vi "Init.vi"(8 "error in (no error)":errorcluster, 9 "Value":string, 10 "Data [value]":T1=enum."value") -> (0 "error out":errorcluster, 3 "Set Query out":refnum<class "Set Query.lvclass">)   [LabVIEW 2013, in "Set Query.lvclass"]
doc: "Copyright 2018, Carya Automatisering, Wiebe Walstra."
uses:
  Set Query.lvclass
  Data.ctl
  Set Query.lvclass/Set Query.ctl
  CConfig Object.lvclass
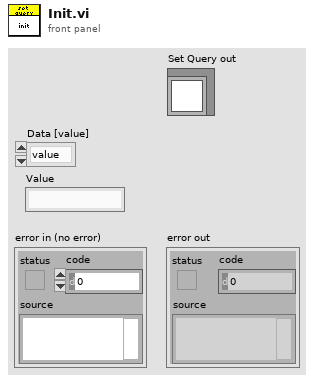
[diagram p1: front panel]
types:
  T1 = typedef "CConfig Object.lvclass/Data.ctl" = enum16{"pre", "name", "middle", "value", "post", "newline", "persistant", "tagged", "type"}
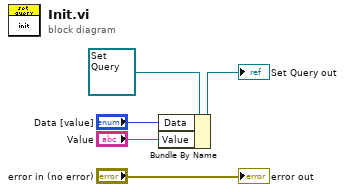
[diagram p0: block diagram]
diagram:
  n1 = Bundle By Name(cluster=refnum<class "Set Query.lvclass"> refnum ("Set Query in"), "Data"="Data [value]", "Value"="Value") -> (→"Set Query out":refnum<class "Set Query.lvclass">)
  "error out" <- "error in (no error)"
